vi "K2231_Output_on_off.vi"(2 "error in (no error)":errorcluster, 3 "Enable Output (T: Enable)":bool=TRUE, 4 "VISA resource name":refnum<visa-resource-name>="K2231A") -> (0 "error out":errorcluster, 1 "VISA resource name out":refnum<visa-resource-name>)   [LabVIEW 2023]
doc: "To make the output power state On/Off for all three channels simultaneously.\n\n* Output Enable (T:Enable) : \n If true it Switches On the power supply Output else doesn't respond."
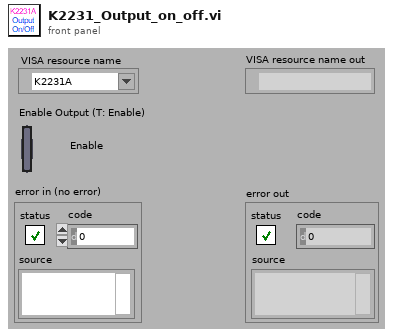
[diagram p1: front panel]
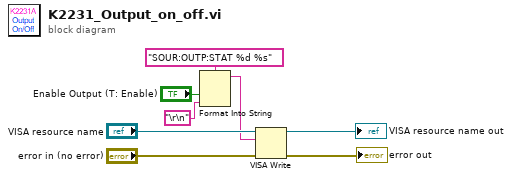
[diagram p0: block diagram]
diagram:
  n1 = Format Into String(format string="SOUR:OUTP:STAT %d %s", "Enable Output (T: Enable)", "\r\n") -> (resulting string=w3:string)  [unwired: 2 in, 1 out]
  n2 = VISA Write(VISA resource name="VISA resource name", write buffer=w3, error in (no error)="error in (no error)") -> (VISA resource name out=→"VISA resource name out":refnum<visa-resource-name>, error out=→"error out":errorcluster)  [unwired: 1 out]
